vi "Rendevous.vi"() -> ()   [LabVIEW 2020]
doc: "Use this template to build a master/slave design pattern. The master loop always executes. It notifies one or more slave loops to execute their code. The slave loop(s) continue executing until they complete, then wait for another notification. Contrast this with the Producer/Consumer pattern in which the consumer loops execute only when they have data in their queue."
panel:
  in  "stop":bool
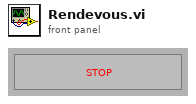
[diagram p1: front panel]
types:
  T1 = typedef "Rendezvous RefNum" = refnum<k1>
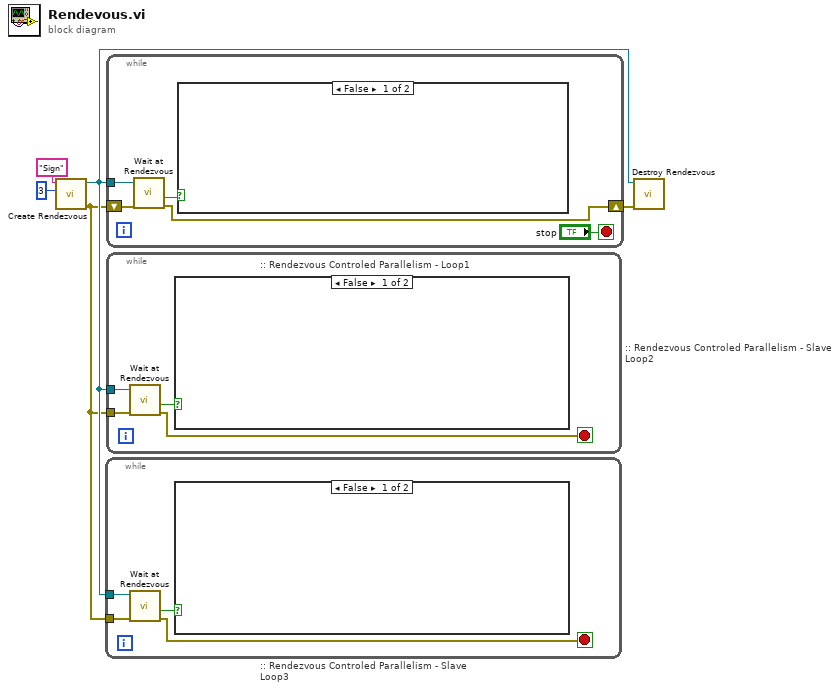
[diagram p0: block diagram]
diagram:
  n1 = call <vilib>:"Create Rendezvous.vi"("size (2)"=3 ("size (1)"), "name (unnamed)"="Sign") -> ("error out"=w1:errorcluster, "rendezvous"=w2:T1)  [unwired: 3 in, 1 out]
  n2 = while ":: Rendezvous Controled Parallelism - Slave Loop3" {
    tunnel: w2 -> [w9]
    tunnel: w1 -> [w8]
    stop <- w7 stop-if-true
    n3 = call <vilib>:"Wait at Rendezvous.vi"("error in (no error)"=w8, "rendezvous"=w9) -> ("error out"=w7:errorcluster, "timed out"=w6:bool)  [unwired: 3 in, 1 out]
    n4 = case shown="False" w6 {
      frame False {
      }
      frame True {
      }
    }
  }
  n5 = while ":: Rendezvous Controled Parallelism - Loop1" {
    shift-right: [w10] -> w4
    shift-left: w1 -> [w13]
    tunnel: w2 -> [w11]
    stop <- "stop" stop-if-true
    n6 = call <vilib>:"Wait at Rendezvous.vi"("error in (no error)"=w13, "rendezvous"=w11) -> ("error out"=w10:errorcluster, "timed out"=w12:bool)  [unwired: 3 in, 1 out]
    n7 = case shown="False" w12 {
      frame False {
      }
      frame True {
      }
    }
  }
  n8 = while ":: Rendezvous Controled Parallelism - Slave Loop2" {
    tunnel: w2 -> [w18]
    tunnel: w1 -> [w17]
    stop <- w16 stop-if-true
    n9 = call <vilib>:"Wait at Rendezvous.vi"("error in (no error)"=w17, "rendezvous"=w18) -> ("error out"=w16:errorcluster, "timed out"=w15:bool)  [unwired: 3 in, 1 out]
    n10 = case shown="False" w15 {
      frame False {
      }
      frame True {
      }
    }
  }
  n11 = call <vilib>:"Destroy Rendezvous.vi"("error in (no error)"=w4, "rendezvous"=w2) -> ()  [unwired: 4 in, 2 out]
